vi "Open.vi"(7 "Allow multiple opens?":bool, 8 "error in (no error)":errorcluster, 10 "Channel Names":tag[](array[tag])) -> (0 "error out":errorcluster, 3 "DO (N Samples) Ref Out":T1)   [LabVIEW 2021, in "DO Block.lvlib"]
doc: "Opens the reference to the digital output block write channel (ConnectorA/DIO1). You must open a reference before you write values."
uses:
  <vilib>/myRIO/Instrument Drivers/Onboard IO/DO Block/DO Block.lvlib
  <vilib>/myRIO/Instrument Drivers/Onboard IO/DO Block/typedefs/DO Block Reference.ctl
  <vilib>/myRIO/Common/Instrument Driver Framework/Utilities/typedefs/myRIO Generic Hardware Reference.ctl
  <vilib>/myRIO/Common/Instrument Driver Framework/Utilities/typedefs/Hardware Version Enum.ctl
  <vilib>/myRIO/Common/Instrument Driver Framework/Utilities/typedefs/myRIO v1.0 Reference.ctl
  <vilib>/myRIO/Common/Instrument Driver Framework/Utilities/typedefs/Generic FPGA Reference.ctl
  <vilib>/myRIO/Common/Instrument Driver Framework/myRIO v1.0/DO Block/typedefs/DO Block Channels List.ctl
  <vilib>/myRIO/Common/Instrument Driver Framework/myRIO v1.0/DO Block/typedefs/DO Block Channels Enum.ctl
  <vilib>/userdefined/High Color/nirio_resource_hc.ctl
panel:
  # "DO (N Samples) Open"
  # "Opens a reference to the myRIO hardware and configures the DO (N Samples) Reference with channels to be written"
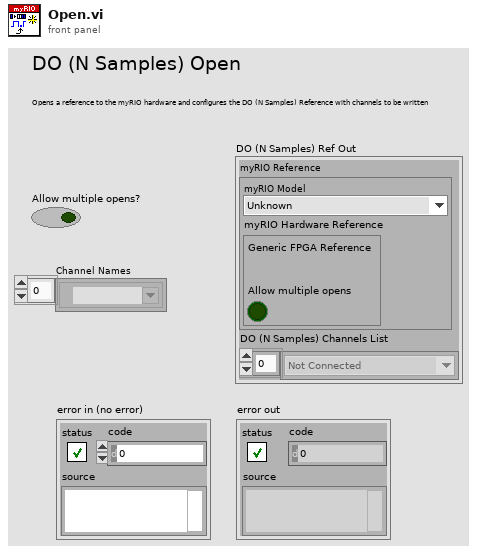
[diagram p1: front panel]
types:
  T1 = typedef "DO Block.lvlib/DO Block Reference.ctl" = cluster{"myRIO Reference":T2, "DO (N Samples) Channels List":T6}
  T2 = typedef "myRIO Generic Hardware Reference.ctl" = cluster{"myRIO Model":T3, "myRIO Hardware Reference":T4}
  T3 = typedef "Hardware Version Enum.ctl" = enum16{"Unknown", "myRIO-1900", "myRIO-1950", "roboRIO", "NI ELVIS RIO CM", "ELVIS III"}
  T4 = typedef "myRIO v1.0 Reference.ctl" = cluster{"Generic FPGA Reference":T5, "Allow multiple opens":bool}
  T5 = typedef "Generic FPGA Reference.ctl" = refnum<k20>
  T6 = typedef "DO Block Channels List.ctl" = T7[]
  T7 = typedef "DO Block Channels Enum.ctl" = enum16{"Not Connected", "A/DO0 (N Samples)", "A/DO1 (N Samples)", "A/DO2 (N Samples)", "A/DO3 (N Samples)", "A/DO4 (N Samples)", "A/DO5 (N Samples)", "A/DO6 (N Samples)", "A/DO7 (N Samples)", "A/DO8 (N Samples)", "A/DO9 (N Samples)", "A/DO10 (N Samples)", "A/DO11 (N Samples)", "A/DO12 (N Samples)", "A/DO13 (N Samples)", "A/DO14 (N Samples)", "A/DO15 (N Samples)", "A/DO16 (N Samples)", "A/DO17 (N Samples)", "A/DO18 (N Samples)", "A/DO19 (N Samples)", "B/DO0 (N Samples)", "B/DO1 (N Samples)", "B/DO2 (N Samples)", "B/DO3 (N Samples)", "B/DO4 (N Samples)", "B/DO5 (N Samples)", "B/DO6 (N Samples)", "B/DO7 (N Samples)", "B/DO8 (N Samples)", "B/DO9 (N Samples)", "B/DO10 (N Samples)", "B/DO11 (N Samples)", "B/DO12 (N Samples)", "B/DO13 (N Samples)", "B/DO14 (N Samples)", "B/DO15 (N Samples)", "B/DO16 (N Samples)", "B/DO17 (N Samples)", "B/DO18 (N Samples)", "B/DO19 (N Samples)"}
  T8 = typedef "nirio_resource_hc.ctl" = tag
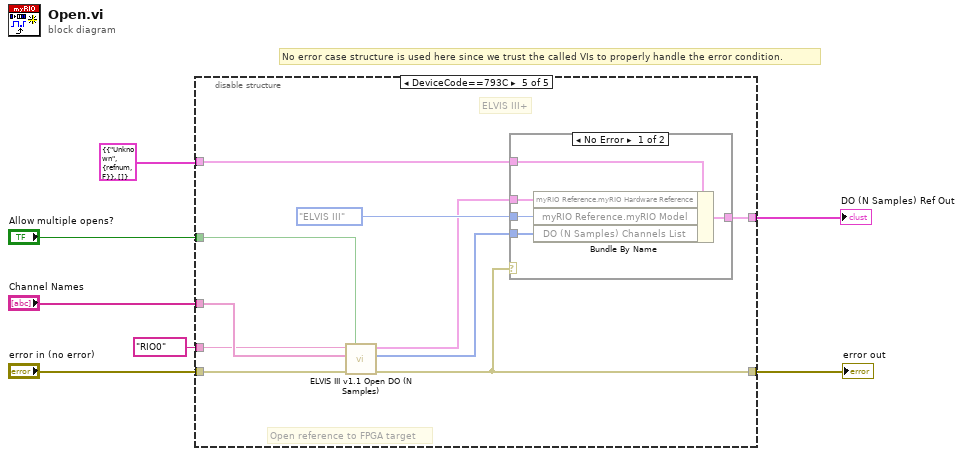
[diagram p0: block diagram]
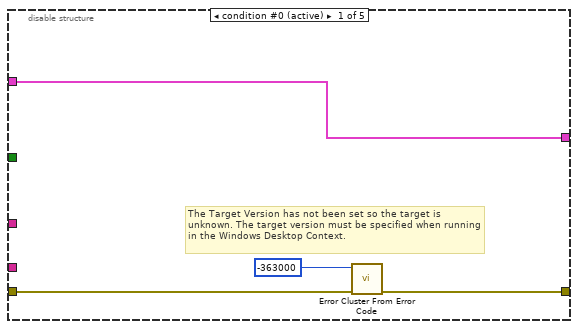
[diagram p2: hidden frame]
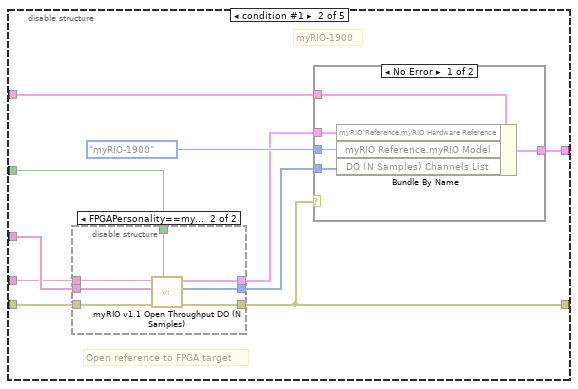
[diagram p3: hidden frame]
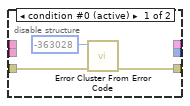
[diagram p4: hidden frame]
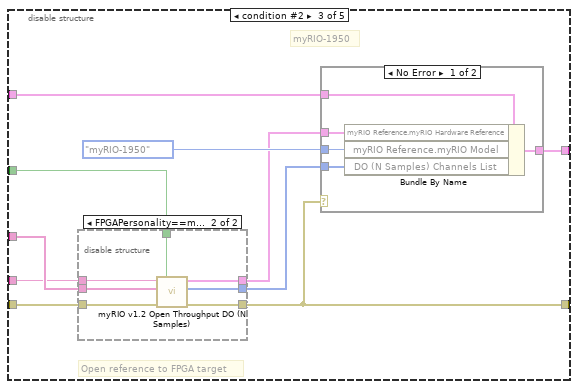
[diagram p6: hidden frame]
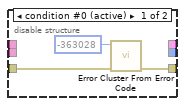
[diagram p7: hidden frame]
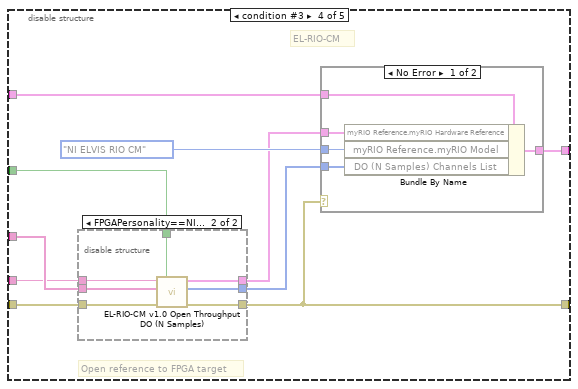
[diagram p9: hidden frame]
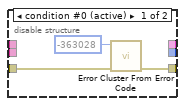
[diagram p10: hidden frame]
diagram:
  # "No error case structure is used here since we trust the called VIs to properly handle the error condition."
  n1 = disable-structure shown="DeviceCode==793C" {
    disable-tunnel: [w11 w13 w40 w66 w91] -> w5
    disable-tunnel: "Channel Names" -> [_ w21 w47 w73 w94]
    disable-tunnel: "Allow multiple opens?" -> [_ w17 w46 w72 w95]
    disable-tunnel: [w8 w20 w45 w71 w90] -> w1
    disable-tunnel: "error in (no error)" -> [w10 w18 w43 w69 w92]
    disable-tunnel: T1 {"myRIO Reference"={"myRIO Model"=enum."Unknown", "myRIO Hardware Reference"={"Generic FPGA Reference"=refnum, "Allow multiple opens"=FALSE}}, "DO (N Samples) Channels List"=[]} ("DO (N Samples) Write Ref Out") -> [w8 w16 w42 w68 w96]
    disable-tunnel: T8 "RIO0" ("Resource name") -> [_ w14 w41 w67 w93]
    frame condition #0 (active) {
      # "The Target Version has not been set so the target is unknown. The target version must be specified when running in the Windows Desktop Context."
      n2 = call <vilib>:"Error Cluster From Error Code.vi"("error in (no error)"=w10, "error code (0)"=-363000) -> ("error out"=w11:errorcluster)  [unwired: 7 in]
    }
    frame condition #1 {
      # "myRIO-1900"
      # "Open reference to FPGA target"
      n3 = disable-structure shown="FPGAPersonality==myRIO_FP_Throughput" {
        disable-tunnel: w21 -> [_ w29]
        disable-tunnel: w18 -> [w23 w28]
        disable-tunnel: w17 -> [_ w31]
        disable-tunnel: [_ w26] -> w15
        disable-tunnel: w14 -> [_ w30]
        disable-tunnel: [w22 w25] -> w13
        disable-tunnel: [_ w27] -> w12
        frame condition #0 (active) {
          n4 = call <vilib>:"Error Cluster From Error Code.vi"("error in (no error)"=w23, "error code (0)"=-363028) -> ("error out"=w22:errorcluster)  [unwired: 7 in]
        }
        frame condition #1 {
          n5 = call <vilib>:"myRIO v1.1 Open Throughput DO (N Samples).vi"("Allow multiple opens?"=w31, "error in (no error)"=w28, "Channel Names"=w29, "Resource name"=w30) -> ("error out"=w25:errorcluster, "DO (N Samples) Channel List"=w26:T6, "myRIO Ref Out"=w27:T4)  [unwired: 5 in]
        }
      }
      n6 = case shown="No Error" w13 {
        tunnel: [w36 w37] -> w20
        tunnel: Hardware_Version_Enum."myRIO-1900" ("Hardware Version Enum") -> [w35 _]
        tunnel: w16 -> [w34 w37]
        tunnel: w15 -> [w33 _]
        tunnel: w12 -> [w32 _]
        frame No Error {
          n7 = Bundle By Name(cluster=w34, "myRIO Reference.myRIO Hardware Reference"=w32, "myRIO Reference.myRIO Model"=w35, "DO (N Samples) Channels List"=w33) -> (w36:T1)
        }
        frame Error {
        }
      }
    }
    frame condition #2 {
      # "myRIO-1950"
      # "Open reference to FPGA target"
      n8 = disable-structure shown="FPGAPersonality==myRIO_FP_Throughput" {
        disable-tunnel: w47 -> [_ w55]
        disable-tunnel: w46 -> [_ w57]
        disable-tunnel: w43 -> [w49 w54]
        disable-tunnel: w41 -> [_ w56]
        disable-tunnel: [w48 w51] -> w40
        disable-tunnel: [_ w53] -> w39
        disable-tunnel: [_ w52] -> w38
        frame condition #0 (active) {
          n9 = call <vilib>:"Error Cluster From Error Code.vi"("error in (no error)"=w49, "error code (0)"=-363028) -> ("error out"=w48:errorcluster)  [unwired: 7 in]
        }
        frame condition #1 {
          n10 = call <vilib>:"myRIO v1.2 Open Throughput DO (N Samples).vi"("Allow multiple opens?"=w57, "error in (no error)"=w54, "Channel Names"=w55, "Resource name"=w56) -> ("error out"=w51:errorcluster, "DO (N Samples) Channel List"=w52:T6, "myRIO Ref Out"=w53:T4)  [unwired: 5 in]
        }
      }
      n11 = case shown="No Error" w40 {
        tunnel: [w62 w63] -> w45
        tunnel: Hardware_Version_Enum."myRIO-1950" ("Hardware Version Enum") -> [w61 _]
        tunnel: w42 -> [w60 w63]
        tunnel: w39 -> [w59 _]
        tunnel: w38 -> [w58 _]
        frame No Error {
          n12 = Bundle By Name(cluster=w60, "myRIO Reference.myRIO Hardware Reference"=w59, "myRIO Reference.myRIO Model"=w61, "DO (N Samples) Channels List"=w58) -> (w62:T1)
        }
        frame Error {
        }
      }
    }
    frame condition #3 {
      # "EL-RIO-CM"
      # "Open reference to FPGA target"
      n13 = disable-structure shown="FPGAPersonality==NI_ELVIS_RIO_CM_FP_Throughput" {
        disable-tunnel: w73 -> [_ w81]
        disable-tunnel: w72 -> [_ w83]
        disable-tunnel: w69 -> [w75 w80]
        disable-tunnel: w67 -> [_ w82]
        disable-tunnel: [w74 w77] -> w66
        disable-tunnel: [_ w79] -> w65
        disable-tunnel: [_ w78] -> w64
        frame condition #0 (active) {
          n14 = call <vilib>:"Error Cluster From Error Code.vi"("error in (no error)"=w75, "error code (0)"=-363028) -> ("error out"=w74:errorcluster)  [unwired: 7 in]
        }
        frame condition #1 {
          n15 = call <vilib>:"EL-RIO-CM v1.0 Open Throughput DO (N Samples).vi"("Allow multiple opens?"=w83, "error in (no error)"=w80, "Channel Names"=w81, "Resource name"=w82) -> ("error out"=w77:errorcluster, "DO (N Samples) Channel List"=w78:T6, "myRIO Ref Out"=w79:T4)  [unwired: 5 in]
        }
      }
      n16 = case shown="No Error" w66 {
        tunnel: [w88 w89] -> w71
        tunnel: Hardware_Version_Enum."NI ELVIS RIO CM" ("Hardware Version Enum") -> [w87 _]
        tunnel: w68 -> [w86 w89]
        tunnel: w65 -> [w85 _]
        tunnel: w64 -> [w84 _]
        frame No Error {
          n17 = Bundle By Name(cluster=w86, "myRIO Reference.myRIO Hardware Reference"=w85, "myRIO Reference.myRIO Model"=w87, "DO (N Samples) Channels List"=w84) -> (w88:T1)
        }
        frame Error {
        }
      }
    }
    frame condition #4 {
      # "ELVIS III+"
      # "Open reference to FPGA target"
      n18 = call <vilib>:"ELVIS III v1.1 Open DO (N Samples).vi"("Allow multiple opens?"=w95, "error in (no error)"=w92, "Channel Names"=w94, "Resource name"=w93) -> ("error out"=w91:errorcluster, "DO (N Samples) Channel List"=w97:T6, "myRIO Ref Out"=w98:T4)  [unwired: 5 in]
      n19 = case shown="No Error" w91 {
        tunnel: [w104 w105] -> w90
        tunnel: Hardware_Version_Enum."ELVIS III" ("Hardware Version Enum") -> [w103 _]
        tunnel: w96 -> [w102 w105]
        tunnel: w98 -> [w101 _]
        tunnel: w97 -> [w100 _]
        frame No Error {
          n20 = Bundle By Name(cluster=w102, "myRIO Reference.myRIO Hardware Reference"=w101, "myRIO Reference.myRIO Model"=w103, "DO (N Samples) Channels List"=w100) -> (w104:T1)
        }
        frame Error {
        }
      }
    }
  }
  "DO (N Samples) Ref Out" <- w1
  "error out" <- w5
